vi "Test_Status.vi"() -> ()   [LabVIEW 2015, in "WordManipulationTests.lvlib"]
uses:
  MotionModuleUtilities/StateMachine.ctl
  WordManipulationTests.lvlib
  async/WordManipulationLibrary.lvlib
panel:
  out "Status":T1[](array[typedef])
  out "WordtoStatus":T1[](array[typedef])
  out "Word":u16[](array[numeric]) format="%08b"
  out "Array":bool[](array[boolean])
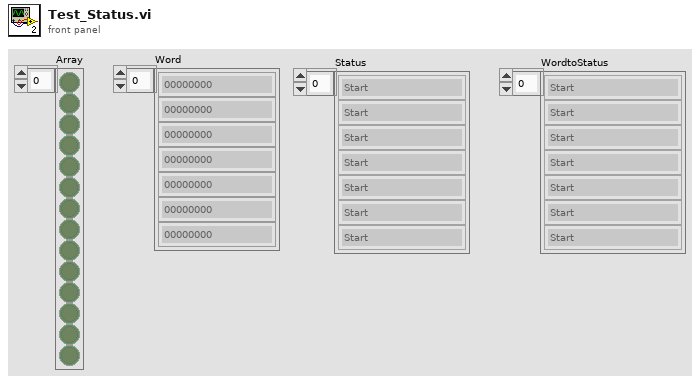
[diagram p1: front panel]
types:
  T1 = typedef "WordManipulationLibrary.lvlib/StateMachine.ctl" = enum16{"Start", "Not Ready to Switch On", "Switch On Disabled", "Ready to Switch On", "Switched On", "Operation enable", "Quick Stop Active", "Fault Reaction Active", "Fault"}
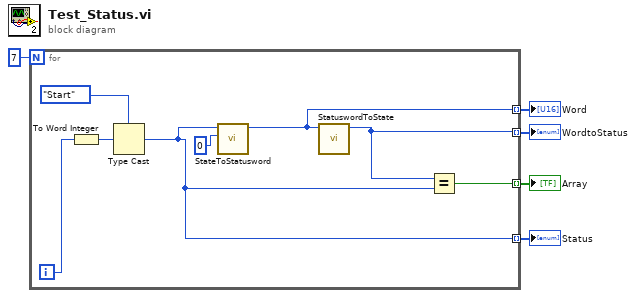
[diagram p0: block diagram]
diagram:
  n1 = for {
    N: 7 -> [_]
    tunnel: [w13] -> w4 mode=indexing
    tunnel: [w7] -> w2 mode=indexing
    tunnel: [w9] -> w1 mode=indexing
    tunnel: [w6] -> w3 mode=indexing
    i -> [w12]
    n2 = To Word Integer(number=w12) -> (16bit integer=w11:i16)
    n3 = Type Cast(type=StateMachine."Start" ("CurrentStatus"), x=w11) -> (*(type *) &x=w9:T1)
    n4 = call "StateToStatusword.vi"("Numeric"=u16 0 ("ControlWord In"), "CurrentStatus"=w9) -> ("StatusWord"=w6:u16)  [unwired: 9 in]
    n5 = call "StatuswordToState.vi"("Data_In"=w6) -> ("Status"=w7:T1)  [unwired: 10 in]
    n6 = Equal?(x=w7, y=w9) -> (x = y?=w13:bool)
  }
  "Array" <- w4
  "Word" <- w3
  "WordtoStatus" <- w2
  "Status" <- w1
